vi "config_file_fgv.vi"(7 "cmd":enum16{"save", "load"}(ring), 8 "error in":errorcluster, 11 "Config":T1={"Lower Cut-Off"=0.5, "Vacuum Trigger level"=20.0, "state settings"={"method"=enum."histogram", "histogram size"=512, "histogram method"=enum."mode", "reserved"=1.0}, "SPA-300 Setting"={"Bonding force (g)"=0.0, "Bonding time (ms)"=512.0, "Pickup force (g)"=0.0, "Pickup time (ms)"=1.0, "Speed"=enum."Slow"}, "sensor file"=path ""} {"state settings"."reserved" format="%0.2f"}) -> (0 "error out":errorcluster, 2 "XML String":string caption="XML 문자열", 3 "var":T1={"Lower Cut-Off"=0.5, "Vacuum Trigger level"=20.0, "state settings"={"method"=enum."histogram", "histogram size"=512, "histogram method"=enum."mode", "reserved"=1.0}, "SPA-300 Setting"={"Bonding force (g)"=0.0, "Bonding time (ms)"=512.0, "Pickup force (g)"=0.0, "Pickup time (ms)"=1.0, "Speed"=enum."Slow"}, "sensor file"=path ""} {"state settings"."reserved" format="%0.2f"})   [LabVIEW 2016]
uses:
  ctl/config_ctl.ctl
  <vilib>/Utility/xml.llb/Write to XML File(string).vi
  <vilib>/Utility/xml.llb/Read From XML File(string).vi
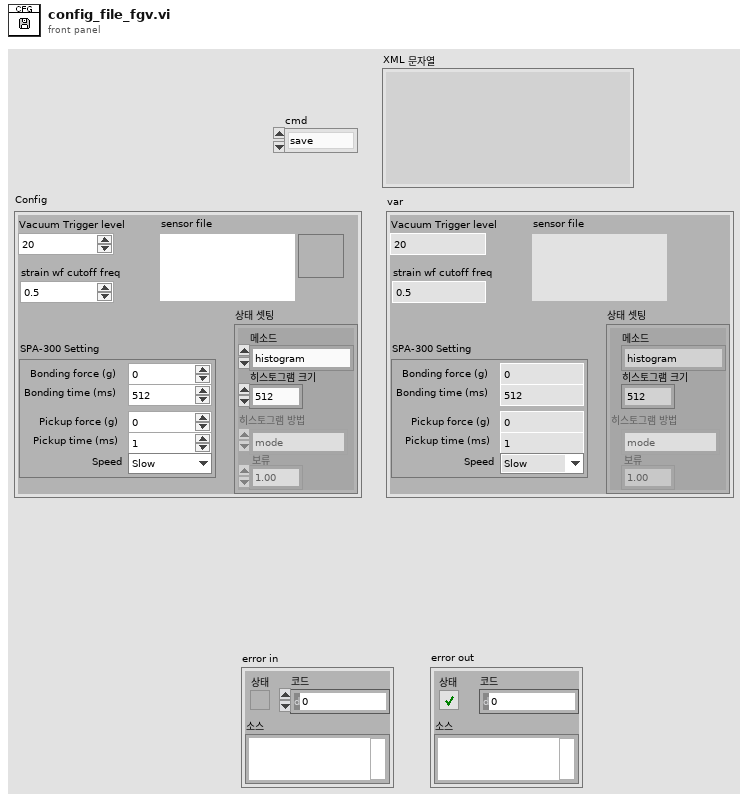
[diagram p1: front panel]
types:
  T1 = typedef "config_ctl.ctl" = cluster{"Lower Cut-Off":dbl, "Vacuum Trigger level":dbl, "state settings":cluster{"method":enum32{"histogram", "peak", "auto select"}, "histogram size":i32, "histogram method":enum16{"mode"}, "reserved":dbl}, "SPA-300 Setting":cluster{"Bonding force (g)":dbl, "Bonding time (ms)":dbl, "Pickup force (g)":dbl, "Pickup time (ms)":dbl, "Speed":enum16{"Slow", "Fast"}}, "sensor file":path}
  T2 = enum16{"open", "replace", "create", "open or create", "replace or create", "replace or create with confirmation"}
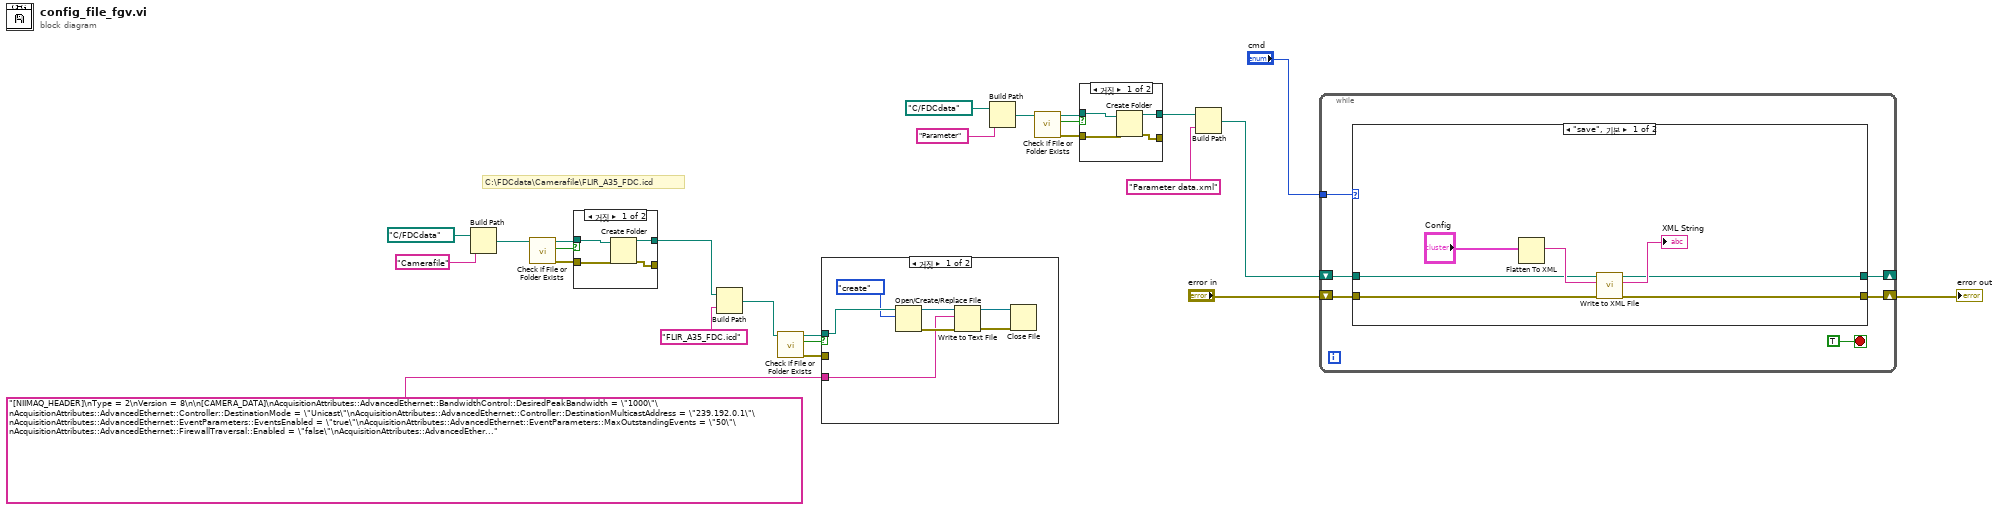
[diagram p0: block diagram]
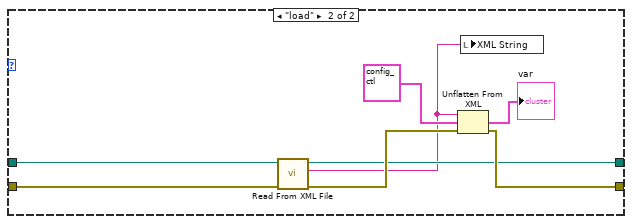
[diagram p5: hidden frame]
diagram:
  # "C:\\FDCdata\\Camerafile\\FLIR_A35_FDC.icd"
  n1 = Build Path(base path=path "C:/FDCdata" ("파일 경로(대화 상자 사용)"), name or relative path="Camerafile" ("이름 또는 상대 경로")) -> (appended path=w15:path)
  n2 = call <vilib>:"Check if File or Folder Exists.vi"("path"=w15) -> ("error out"=w14:errorcluster, "file or folder exists?"=w13:bool, "dup path"=w12:path)  [unwired: 8 in]
  n3 = case shown="거짓" w13 {
    tunnel: w12 -> [w29 w31]
    tunnel: w14 -> [w28 w30]
    tunnel: [w27 w31] -> w8
    tunnel: [w26 w30] -> _
    frame False {
      n4 = Create Folder(path (use dialog)=w29, error in=w28) -> (created path=w27:path, error out=w26:errorcluster)  [unwired: 1 in, 1 out]
    }
    frame True {
    }
  }
  n5 = Build Path(base path=w8, name or relative path="FLIR_A35_FDC.icd" ("이름 또는 상대 경로")) -> (appended path=w4:path)
  n6 = call <vilib>:"Check if File or Folder Exists.vi"("path"=w4) -> ("error out"=w5:errorcluster, "file or folder exists?"=w6:bool, "dup path"=w7:path)  [unwired: 8 in]
  n7 = case shown="거짓" w6 {
    tunnel: w7 -> [w38 _]
    tunnel: w5 -> [_ _]
    tunnel: "[NIIMAQ_HEADER]\nType = 2\nVersion = 8\n\n[CAMERA_DATA]\nAcquisitionAttributes::AdvancedEthernet::BandwidthControl::DesiredPeakBandwidth = \"1000\"\nAcquisitionAttributes::AdvancedEthernet::Controller::DestinationMode = \"Unicast\"\nAcquisitionAttributes::AdvancedEthernet::Controller::DestinationMulticastAddress = \"239.192.0.1\"\nAcquisitionAttributes::AdvancedEthernet::EventParameters::EventsEnabled = \"true\"\nAcquisitionAttributes::AdvancedEthernet::EventParameters::MaxOutstandingEvents = \"50\"\nAcquisitionAttributes::AdvancedEthernet::FirewallTraversal::Enabled = \"false\"\nAcquisitionAttributes::AdvancedEthernet::FirewallTraversal::KeepAliveTime = \"30\"\nAcquisitionAttributes::AdvancedEthernet::LostPacketMode = \"Ignore\"\nAcquisitionAttributes::AdvancedEthernet::ResendParameters::MaxResendsPerPacket = \"25\"\nAcquisitionAttributes::AdvancedEthernet::ResendParameters::MemoryWindowSize = \"1024\"\nAcquisitionAttributes::AdvancedEthernet::ResendParameters::MissingPacketTimeout = \"2\"\nAcquisitionAttributes::AdvancedEthernet::ResendParameters::NewPacketTimeout = \"100\"\nAcquisitionAttributes::AdvancedEthernet::ResendParameters::ResendBatchingPercentage = \"10\"\nAcquisitionAttributes::AdvancedEthernet::ResendParameters::ResendResponseTimeout = \"2\"\nAcquisitionAttributes::AdvancedEthernet::ResendParameters::ResendsEnabled = \"true\"\nAcquisitionAttributes::AdvancedEthernet::ResendParameters::ResendThresholdPercentage = \"5\"\nAcquisitionAttributes::AdvancedEthernet::ResendParameters::ResendTimerResolution = \"1\"\nAcquisitionAttributes::AdvancedEthernet::TestPacketParameters::MaxTestPacketRetries = \"1\"\nAcquisitionAttributes::AdvancedEthernet::TestPacketParameters::TestPacketEnabled = \"true\"\nAcquisitionAttributes::AdvancedEthernet::TestPacketParameters::TestPacketTimeout = \"250\"\nAcquisitionAttributes::AdvancedGenicam::CommandTimeout = \"100\"\nAcquisitionAttributes::Bayer::Algorithm = \"Bilinear\"\nAcquisitionAttributes::Bayer::GainB = \"1\"\nAcquisitionAttributes::Bayer::GainG = \"1\"\nAcquisitionAttributes::Bayer::GainR = \"1\"\nAcquisitionAttributes::Bayer::Pattern = \"Use hardware value\"\nAcquisitionAttributes::BitsPerPixel = \"Use hardware value\"\nAcquisitionAttributes::ChunkDataDecoding::ChunkDataDecodingEnabled = \"false\"\nAcquisitionAttributes::ChunkDataDecoding::MaximumChunkCopySize = \"64\"\nAcquisitionAttributes::IgnoreFirstFrame = \"false\"\nAcquisitionAttributes::ImageDecoderCopyMode = \"Auto\"\nAcquisitionAttributes::OutputImageType = \"Auto\"\nAcquisitionAttributes::OverwriteMode = \"Get Newest\"\nAcquisitionAttributes::PacketSize = \"1000\"\nAcquisitionAttributes::PixelSignedness = \"Signed\"\nAcquisitionAttributes::ReceiveTimestampMode = \"None\"\nAcquisitionAttributes::ShiftPixelBits = \"false\"\nAcquisitionAttributes::SwapPixelBytes = \"false\"\nAcquisitionAttributes::Timeout = \"5000\"\nCameraAttributes::AcquisitionControl::AcquisitionFrameCount = \"1\"\nCameraAttributes::AcquisitionControl::AcquisitionMode = \"Continuous\"\nCameraAttributes::CameraControl::BaudRate = \"baudAuto\"\nCameraAttributes::CameraControl::CorrectionMask = \"575\"\nCameraAttributes::CameraControl::IgnoreCRC = \"On\"\nCameraAttributes::CameraControl::NUCMode = \"Automatic\"\nCameraAttributes::CameraControl::SensorDDEIndex = \"17\"\nCameraAttributes::CameraControl::SensorDDEMode = \"Automatic\"\nCameraAttributes::CameraControl::SensorGainMode = \"LowGainMode\"\nCameraAttributes::CameraControl::ShutterPosition = \"Open\"\nCameraAttributes::CounterAndTimerControl::CounterSelector = \"Counter1\"\nCameraAttributes::CounterAndTimerControl::CounterDecrementEventSource = \"Off\"\nCameraAttributes::CounterAndTimerControl::CounterDuration = \"0\"\nCameraAttributes::CounterAndTimerControl::CounterEventSource = \"Off\"\nCameraAttributes::CounterAndTimerControl::CounterResetActivation = \"Off\"\nCameraAttributes::CounterAndTimerControl::CounterResetSource = \"PLC_Q3\"\nCameraAttributes::CounterAndTimerControl::CounterTriggerSource = \"Off\"\nCameraAttributes::CounterAndTimerControl::CounterValue = \"0\"\nCameraAttributes::CounterAndTimerControl::TimerSelector = \"Timer1\"\nCameraAttributes::CounterAndTimerControl::TimerDelayRaw = \"1024\"\nCameraAttributes::CounterAndTimerControl::TimerDurationRaw = \"4096\"\nCameraAttributes::CounterAndTimerControl::TimerGranularityFactor = \"0\"\nCameraAttributes::CounterAndTimerControl::TimerTriggerActivation = \"RisingEdge\"\nCameraAttributes::CounterAndTimerControl::TimerTriggerSource = \"PLC_Q\"\nCameraAttributes::CounterAndTimerControl::TimerSelector = \"Timer2\"\nCameraAttributes::CounterAndTimerControl::TimerDelayRaw = \"1024\"\nCameraAttributes::CounterAndTimerControl::TimerDurationRaw = \"4096\"\nCameraAttributes::CounterAndTimerControl::TimerGranularityFactor = \"0\"\nCameraAttributes::CounterAndTimerControl::TimerTriggerActivation = \"RisingEdge\"\nCameraAttributes::CounterAndTimerControl::TimerTriggerSource = \"PLC_Q\"\nCameraAttributes::CounterAndTimerControl::TimerSelector = \"Timer3\"\nCameraAttributes::CounterAndTimerControl::TimerDelayRaw = \"1024\"\nCameraAttributes::CounterAndTimerControl::TimerDurationRaw = \"4096\"\nCameraAttributes::CounterAndTimerControl::TimerGranularityFactor = \"0\"\nCameraAttributes::CounterAndTimerControl::TimerTriggerActivation = \"RisingEdge\"\nCameraAttributes::CounterAndTimerControl::TimerTriggerSource = \"PLC_Q\"\nCameraAttributes::CounterAndTimerControl::TimerSelector = \"Timer4\"\nCameraAttributes::CounterAndTimerControl::TimerDelayRaw = \"1024\"\nCameraAttributes::CounterAndTimerControl::TimerDurationRaw = \"4096\"\nCameraAttributes::CounterAndTimerControl::TimerGranularityFactor = \"0\"\nCameraAttributes::CounterAndTimerControl::TimerTriggerActivation = \"RisingEdge\"\nCameraAttributes::CounterAndTimerControl::TimerTriggerSource = \"PLC_Q\"\nCameraAttributes::CounterAndTimerControl::TimerSelector = \"Timer1\"\nCameraAttributes::DeviceControl::DeviceScanType = \"Areascan\"\nCameraAttributes::DigitalIOControl::LineSelector = \"Line0\"\nCameraAttributes::DigitalIOControl::LineDebounceFactor = \"0\"\nCameraAttributes::DigitalIOControl::SyncMode = \"Disabled\"\nCameraAttributes::DigitalIOControl::UserOutputSelector = \"UserOutput0\"\nCameraAttributes::DigitalIOControl::UserOutputValue = \"true\"\nCameraAttributes::EventControl::EventSelector = \"PLC_Interrupt_FIFO0_Q15\"\nCameraAttributes::EventControl::EventNotification = \"On\"\nCameraAttributes::EventControl::EventSelector = \"PLC_Interrupt_FIFO0_Q3\"\nCameraAttributes::EventControl::EventNotification = \"Off\"\nCameraAttributes::EventControl::EventSelector = \"PLC_Interrupt_FIFO0_Q7\"\nCameraAttributes::EventControl::EventNotification = \"Off\"\nCameraAttributes::EventControl::EventSelector = \"PLC_Interrupt_FIFO0_Q10\"\nCameraAttributes::EventControl::EventNotification = \"Off\"\nCameraAttributes::EventControl::EventSelector = \"IPEngineCamHeadSerialComLog\"\nCameraAttributes::EventControl::EventNotification = \"Off\"\nCameraAttributes::EventControl::EventSelector = \"IPEngineCamHeadSerialComLog\"\nCameraAttributes::ImageFormatControl::BinningHorizontal = \"1\"\nCameraAttributes::ImageFormatControl::BinningVertical = \"1\"\nCameraAttributes::ImageFormatControl::DecimationHorizontal = \"1\"\nCameraAttributes::ImageFormatControl::DecimationVertical = \"1\"\nCameraAttributes::ImageFormatControl::Height = \"256\"\nCameraAttributes::ImageFormatControl::OffsetX = \"0\"\nCameraAttributes::ImageFormatControl::OffsetY = \"0\"\nCameraAttributes::ImageFormatControl::PixelFormat = \"Mono16\"\nCameraAttributes::ImageFormatControl::SensorDigitizationTaps = \"One\"\nCameraAttributes::ImageFormatControl::TestImageSelector = \"Off\"\nCameraAttributes::ImageFormatControl::Width = \"320\"\nCameraAttributes::ImageStreamControl::CMOSBitDepth = \"bit14bit\"\nCameraAttributes::ImageStreamControl::DigitalOutput = \"bit14bit\"\nCameraAttributes::ImageStreamControl::IRTestPattern = \"Off\"\nCameraAttributes::ImageStreamControl::LVDSBitDepth = \"bit14bit\"\nCameraAttributes::ImageStreamControl::LVDSMode = \"Disabled\"\nCameraAttributes::ImageStreamControl::XPMode = \"CMOS\"\nCameraAttributes::IPEngine::Grabber::Channel0::AcquisitionConfiguration::GrbCh0AcqCfgIncludeMetadataInImage = \"false\"\nCameraAttributes::IPEngine::Grabber::Channel0::AcquisitionConfiguration::GrbCh0AcqCfgInvertPixelData = \"false\"\nCameraAttributes::IPEngine::Grabber::Channel0::AcquisitionConfiguration::GrbCh0AcqCfgMemoryWaterLevel = \"Level75\"\nCameraAttributes::IPEngine::Grabber::Channel0::AcquisitionConfiguration::GrbCh0AcqCfgPixelBusDataPortMapping = \"CBA\"\nCameraAttributes::IPEngine::Grabber::Channel0::TriggerConfiguration::GrbCh0TrigCfgAutomaticInternalRetrigger = \"false\"\nCameraAttributes::IPEngine::Grabber::Channel0::TriggerConfiguration::GrbCh0TrigCfgContinuousPipeCount = \"Two\"\nCameraAttributes::IPEngine::Grabber::Channel0::TriggerConfiguration::GrbCh0TrigCfgFrameToSkip = \"0\"\nCameraAttributes::IPEngine::Grabber::Channel0::TriggerConfiguration::GrbCh0TrigCfgPLCTriggerable = \"false\"\nCameraAttributes::IPEngine::Grabber::Channel0Extension::GrabberMetadata::GrbCh0MetadataInsertionMode = \"FirstFourBytesOfFirstAcquiredLine\"\nCameraAttributes::IPEngine::Grabber::Channel0Extension::GrabberMetadata::GrbCh0MetadataMsbOverride = \"NotOverriden\"\nCameraAttributes::IPEngine::Grabber::Channel0Extension::GrabberMetadata::GrbCh0MetadataSourceSelection = \"BlockID\"\nCameraAttributes::IPEngine::PortCommunication::Uart0::Uart0BaudRate = \"Baud57600\"\nCameraAttributes::IPEngine::PortCommunication::Uart0::Uart0BaudRateFactor = \"1\"\nCameraAttributes::IPEngine::PortCommunication::Uart0::Uart0BreakDetection = \"true\"\nCameraAttributes::IPEngine::PortCommunication::Uart0::Uart0BreakGeneration = \"true\"\nCameraAttributes::IPEngine::PortCommunication::Uart0::Uart0Loopback = \"false\"\nCameraAttributes::IPEngine::PortCommunication::Uart0::Uart0NumOfStopBits = \"One\"\nCameraAttributes::IPEngine::PortCommunication::Uart0::Uart0Parity = \"None\"\nCameraAttributes::IPEngine::PortCommunication::Uart0::Uart0ReadyToReceive = \"true\"\nCameraAttributes::IPEngine::PortCommunication::Uart1::Uart1BaudRate = \"Baud9600\"\nCameraAttributes::IPEngine::PortCommunication::Uart1::Uart1BaudRateFactor = \"1\"\nCameraAttributes::IPEngine::PortCommunication::Uart1::Uart1BreakDetection = \"false\"\nCameraAttributes::IPEngine::PortCommunication::Uart1::Uart1BreakGeneration = \"false\"\nCameraAttributes::IPEngine::PortCommunication::Uart1::Uart1Loopback = \"false\"\nCameraAttributes::IPEngine::PortCommunication::Uart1::Uart1NumOfStopBits = \"One\"\nCameraAttributes::IPEngine::PortCommunication::Uart1::Uart1Parity = \"None\"\nCameraAttributes::IPEngine::PortCommunication::Uart1::Uart1ReadyToReceive = \"false\"\nCameraAttributes::IPEngine::ProgrammableLogicController::ControlBits::PLC_ctrl0 = \"true\"\nCameraAttributes::IPEngine::ProgrammableLogicController::ControlBits::PLC_ctrl1 = \"false\"\nCameraAttributes::IPEngine::ProgrammableLogicController::ControlBits::PLC_ctrl2 = \"false\"\nCameraAttributes::IPEngine::ProgrammableLogicController::ControlBits::PLC_ctrl3 = \"false\"\nCameraAttributes::IPEngine::ProgrammableLogicController::EnhancedFunctionBlock::CounterTriggerGenerator::PLC_ts_trig0_Enable = \"false\"\nCameraAttributes::IPEngine::ProgrammableLogicController::EnhancedFunctionBlock::CounterTriggerGenerator::PLC_ts_trig1_Enable = \"false\"\nCameraAttributes::IPEngine::ProgrammableLogicController::EnhancedFunctionBlock::CounterTriggerGenerator::PLC_ts_trig2_Enable = \"false\"\nCameraAttributes::IPEngine::ProgrammableLogicController::EnhancedFunctionBlock::CounterTriggerGenerator::PLC_ts_trig3_Enable = \"false\"\nCameraAttributes::IPEngine::ProgrammableLogicController::EnhancedFunctionBlock::CounterTriggerGenerator::PLC_ts_trig_CounterSelect = \"GevTimestampValueLow\"\nCameraAttributes::IPEngine::ProgrammableLogicController::EnhancedFunctionBlock::CounterTriggerGenerator::PLC_ts_trig_Time = \"0\"\nCameraAttributes::IPEngine::ProgrammableLogicController::EnhancedFunctionBlock::Delayer0::PLC_del0_DelayCount = \"1\"\nCameraAttributes::IPEngine::ProgrammableLogicController::EnhancedFunctionBlock::Delayer0::PLC_del0_InputSignal = \"PLC_Q3\"\nCameraAttributes::IPEngine::ProgrammableLogicController::EnhancedFunctionBlock::Delayer0::PLC_del0_ReferenceTimingSignal = \"PLC_rsl0_out\"\nCameraAttributes::IPEngine::ProgrammableLogicController::EnhancedFunctionBlock::Rescaler0::PLC_rsl0_BackupEnabled = \"false\"\nCameraAttributes::IPEngine::ProgrammableLogicController::EnhancedFunctionBlock::Rescaler0::PLC_rsl0_BackupInputSignal = \"Timer1Out\"\nCameraAttributes::IPEngine::ProgrammableLogicController::EnhancedFunctionBlock::Rescaler0::PLC_rsl0_BackupSwitchoverDelay = \"0\"\nCameraAttributes::IPEngine::ProgrammableLogicController::EnhancedFunctionBlock::Rescaler0::PLC_rsl0_Divider = \"256\"\nCameraAttributes::IPEngine::ProgrammableLogicController::EnhancedFunctionBlock::Rescaler0::PLC_rsl0_Granularity = \"OneSystemClockCycle\"\nCameraAttributes::IPEngine::ProgrammableLogicController::EnhancedFunctionBlock::Rescaler0::PLC_rsl0_InputSignal = \"PLC_Q3\"\nCameraAttributes::IPEngine::ProgrammableLogicController::EnhancedFunctionBlock::Rescaler0::PLC_rsl0_Multiplier = \"FrequencyX256\"\nCameraAttributes::IPEngine::ProgrammableLogicController::LookupTable::Q0::PLC_Q0_Operator0 = \"Or\"\nCameraAttributes::IPEngine::ProgrammableLogicController::LookupTable::Q0::PLC_Q0_Operator1 = \"Or\"\nCameraAttributes::IPEngine::ProgrammableLogicController::LookupTable::Q0::PLC_Q0_Operator2 = \"Or\"\nCameraAttributes::IPEngine::ProgrammableLogicController::LookupTable::Q0::PLC_Q0_Variable0 = \"PLC_I5\"\nCameraAttributes::IPEngine::ProgrammableLogicController::LookupTable::Q0::PLC_Q0_Variable1 = \"Zero\"\nCameraAttributes::IPEngine::ProgrammableLogicController::LookupTable::Q0::PLC_Q0_Variable2 = \"Zero\"\nCameraAttributes::IPEngine::ProgrammableLogicController::LookupTable::Q0::PLC_Q0_Variable3 = \"Zero\"\nCameraAttributes::IPEngine::ProgrammableLogicController::LookupTable::Q10::PLC_Q10_Operator0 = \"Or\"\nCameraAttributes::IPEngine::ProgrammableLogicController::LookupTable::Q10::PLC_Q10_Operator1 = \"Or\"\nCameraAttributes::IPEngine::ProgrammableLogicController::LookupTable::Q10::PLC_Q10_Operator2 = \"Or\"\nCameraAttributes::IPEngine::ProgrammableLogicController::LookupTable::Q10::PLC_Q10_Variable0 = \"Zero\"\nCameraAttributes::IPEngine::ProgrammableLogicController::LookupTable::Q10::PLC_Q10_Variable1 = \"Zero\"\nCameraAttributes::IPEngine::ProgrammableLogicController::LookupTable::Q10::PLC_Q10_Variable2 = \"Zero\"\nCameraAttributes::IPEngine::ProgrammableLogicController::LookupTable::Q10::PLC_Q10_Variable3 = \"Zero\"\nCameraAttributes::IPEngine::ProgrammableLogicController::LookupTable::Q11::PLC_Q11_Operator0 = \"Or\"\nCameraAttributes::IPEngine::ProgrammableLogicController::LookupTable::Q11::PLC_Q11_Operator1 = \"Or\"\nCameraAttributes::IPEngine::ProgrammableLogicController::LookupTable::Q11::PLC_Q11_Operator2 = \"Or\"\nCameraAttributes::IPEngine::ProgrammableLogicController::LookupTable::Q11::PLC_Q11_Variable0 = \"Zero\"\nCameraAttributes::IPEngine::ProgrammableLogicController::LookupTable::Q11::PLC_Q11_Variable1 = \"Zero\"\nCameraAttributes::IPEngine::ProgrammableLogicController::LookupTable::Q11::PLC_Q11_Variable2 = \"Zero\"\nCameraAttributes::IPEngine::ProgrammableLogicController::LookupTable::Q11::PLC_Q11_Variable3 = \"Zero\"\nCameraAttributes::IPEngine::ProgrammableLogicController::LookupTable::Q12::PLC_Q12_Operator0 = \"Or\"\nCameraAttributes::IPEngine::ProgrammableLogicController::LookupTable::Q12::PLC_Q12_Operator1 = \"Or\"\nCameraAttributes::IPEngine::ProgrammableLogicController::LookupTable::Q12::PLC_Q12_Operator2 = \"Or\"\nCameraAttributes::IPEngine::ProgrammableLogicController::LookupTable::Q12::PLC_Q12_Variable0 = \"Zero\"\nCameraAttributes::IPEngine::ProgrammableLogicController::LookupTable::Q12::PLC_Q12_Variable1 = \"Zero\"\nCameraAttributes::IPEngine::ProgrammableLogicController::LookupTable::Q12::PLC_Q12_Variable2 = \"Zero\"\nCameraAttributes::IPEngine::ProgrammableLogicController::LookupTable::Q12::PLC_Q12_Variable3 = \"Zero\"\nCameraAttributes::IPEngine::ProgrammableLogicController::LookupTable::Q13::PLC_Q13_Operator0 = \"Or\"\nCameraAttributes::IPEngine::ProgrammableLogicController::LookupTable::Q13::PLC_Q13_Operator1 = \"Or\"\nCameraAttributes::IPEngine::ProgrammableLogicController::LookupTable::Q13::PLC_Q13_Operator2 = \"Or\"\nCameraAttributes::IPEngine::ProgrammableLogicController::LookupTable::Q13::PLC_Q13_Variable0 = \"Zero\"\nCameraAttributes::IPEngine::ProgrammableLogicController::LookupTable::Q13::PLC_Q13_Variable1 = \"Zero\"\nCameraAttributes::IPEngine::ProgrammableLogicController::LookupTable::Q13::PLC_Q13_Variable2 = \"Zero\"\nCameraAttributes::IPEngine::ProgrammableLogicController::LookupTable::Q13::PLC_Q13_Variable3 = \"Zero\"\nCameraAttributes::IPEngine::ProgrammableLogicController::LookupTable::Q14::PLC_Q14_Operator0 = \"Or\"\nCameraAttributes::IPEngine::ProgrammableLogicController::LookupTable::Q14::PLC_Q14_Operator1 = \"Or\"\nCameraAttributes::IPEngine::ProgrammableLogicController::LookupTable::Q14::PLC_Q14_Operator2 = \"Or\"\nCameraAttributes::IPEngine::ProgrammableLogicController::LookupTable::Q14::PLC_Q14_Variable0 = \"Zero\"\nCameraAttributes::IPEngine::ProgrammableLogicController::LookupTable::Q14::PLC_Q14_Variable1 = \"Zero\"\nCameraAttributes::IPEngine::ProgrammableLogicController::LookupTable::Q14::PLC_Q14_Variable2 = \"Zero\"\nCameraAttributes::IPEngine::ProgrammableLogicController::LookupTable::Q14::PLC_Q14_Variable3 = \"Zero\"\nCameraAttributes::IPEngine::ProgrammableLogicController::LookupTable::Q15::PLC_Q15_Operator0 = \"Or\"\nCameraAttributes::IPEngine::ProgrammableLogicController::LookupTable::Q15::PLC_Q15_Operator1 = \"Or\"\nCameraAttributes::IPEngine::ProgrammableLogicController::LookupTable::Q15::PLC_Q15_Operator2 = \"Or\"\nCameraAttributes::IPEngine::ProgrammableLogicController::LookupTable::Q15::PLC_Q15_Variable0 = \"Zero\"\nCameraAttributes::IPEngine::ProgrammableLogicController::LookupTable::Q15::PLC_Q15_Variable1 = \"Zero\"\nCameraAttributes::IPEngine::ProgrammableLogicController::LookupTable::Q15::PLC_Q15_Variable2 = \"Zero\"\nCameraAttributes::IPEngine::ProgrammableLogicController::LookupTable::Q15::PLC_Q15_Variable3 = \"Zero\"\nCameraAttributes::IPEngine::ProgrammableLogicController::LookupTable::Q16::PLC_Q16_Operator0 = \"Or\"\nCameraAttributes::IPEngine::ProgrammableLogicController::LookupTable::Q16::PLC_Q16_Operator1 = \"Or\"\nCameraAttributes::IPEngine::ProgrammableLogicController::LookupTable::Q16::PLC_Q16_Operator2 = \"Or\"\nCameraAttributes::IPEngine::ProgrammableLogicController::LookupTable::Q16::PLC_Q16_Variable0 = \"Zero\"\nCameraAttributes::IPEngine::ProgrammableLogicController::LookupTable::Q16::PLC_Q16_Variable1 = \"Zero\"\nCameraAttributes::IPEngine::ProgrammableLogicController::LookupTable::Q16::PLC_Q16_Variable2 = \"Zero\"\nCameraAttributes::IPEngine::ProgrammableLogicController::LookupTable::Q16::PLC_Q16_Variable3 = \"Zero\"\nCameraAttributes::IPEngine::ProgrammableLogicController::LookupTable::Q17::PLC_Q17_Operator0 = \"Or\"\nCameraAttributes::IPEngine::ProgrammableLogicController::LookupTable::Q17::PLC_Q17_Operator1 = \"Or\"\nCameraAttributes::IPEngine::ProgrammableLogicController::LookupTable::Q17::PLC_Q17_Operator2 = \"Or\"\nCameraAttributes::IPEngine::ProgrammableLogicController::LookupTable::Q17::PLC_Q17_Variable0 = \"Zero\"\nCameraAttributes::IPEngine::ProgrammableLogicController::LookupTable::Q17::PLC_Q17_Variable1 = \"Zero\"\nCameraAttributes::IPEngine::ProgrammableLogicController::LookupTable::Q17::PLC_Q17_Variable2 = \"Zero\"\nCameraAttributes::IPEngine::ProgrammableLogicController::LookupTable::Q17::PLC_Q17_Variable3 = \"Zero\"\nCameraAttributes::IPEngine::ProgrammableLogicController::LookupTable::Q1::PLC_Q1_Operator0 = \"Or\"\nCameraAttributes::IPEngine::ProgrammableLogicController::LookupTable::Q1::PLC_Q1_Operator1 = \"Or\"\nCameraAttributes::IPEngine::ProgrammableLogicController::LookupTable::Q1::PLC_Q1_Operator2 = \"Or\"\nCameraAttributes::IPEngine::ProgrammableLogicController::LookupTable::Q1::PLC_Q1_Variable0 = \"Zero\"\nCameraAttributes::IPEngine::ProgrammableLogicController::LookupTable::Q1::PLC_Q1_Variable1 = \"Zero\"\nCameraAttributes::IPEngine::ProgrammableLogicController::LookupTable::Q1::PLC_Q1_Variable2 = \"Zero\"\nCameraAttributes::IPEngine::ProgrammableLogicController::LookupTable::Q1::PLC_Q1_Variable3 = \"Zero\"\nCameraAttributes::IPEngine::ProgrammableLogicController::LookupTable::Q2::PLC_Q2_Operator0 = \"Or\"\nCameraAttributes::IPEngine::ProgrammableLogicController::LookupTable::Q2::PLC_Q2_Operator1 = \"Or\"\nCameraAttributes::IPEngine::ProgrammableLogicController::LookupTable::Q2::PLC_Q2_Operator2 = \"Or\"\nCameraAttributes::IPEngine::ProgrammableLogicController::LookupTable::Q2::PLC_Q2_Variable0 = \"PLC_I1\"\nCameraAttributes::IPEngine::ProgrammableLogicController::LookupTable::Q2::PLC_Q2_Variable1 = \"Zero\"\nCameraAttributes::IPEngine::ProgrammableLogicController::LookupTable::Q2::PLC_Q2_Variable2 = \"Zero\"\nCameraAttributes::IPEngine::ProgrammableLogicController::LookupTable::Q2::PLC_Q2_Variable3 = \"Zero\"\nCameraAttributes::IPEngine::ProgrammableLogicController::LookupTable::Q3::PLC_Q3_Operator0 = \"Or\"\nCameraAttributes::IPEngine::ProgrammableLogicController::LookupTable::Q3::PLC_Q3_Operator1 = \"Or\"\nCameraAttributes::IPEngine::ProgrammableLogicController::LookupTable::Q3::PLC_Q3_Operator2 = \"Or\"\nCameraAttributes::IPEngine::ProgrammableLogicController::LookupTable::Q3::PLC_Q3_Variable0 = \"One\"\nCameraAttributes::IPEngine::ProgrammableLogicController::LookupTable::Q3::PLC_Q3_Variable1 = \"Zero\"\nCameraAttributes::IPEngine::ProgrammableLogicController::LookupTable::Q3::PLC_Q3_Variable2 = \"Zero\"\nCameraAttributes::IPEngine::ProgrammableLogicController::LookupTable::Q3::PLC_Q3_Variable3 = \"Zero\"\nCameraAttributes::IPEngine::ProgrammableLogicController::LookupTable::Q4::PLC_Q4_Operator0 = \"Or\"\nCameraAttributes::IPEngine::ProgrammableLogicController::LookupTable::Q4::PLC_Q4_Operator1 = \"Or\"\nCameraAttributes::IPEngine::ProgrammableLogicController::LookupTable::Q4::PLC_Q4_Operator2 = \"Or\"\nCameraAttributes::IPEngine::ProgrammableLogicController::LookupTable::Q4::PLC_Q4_Variable0 = \"Zero\"\nCameraAttributes::IPEngine::ProgrammableLogicController::LookupTable::Q4::PLC_Q4_Variable1 = \"Zero\"\nCameraAttributes::IPEngine::ProgrammableLogicController::LookupTable::Q4::PLC_Q4_Variable2 = \"Zero\"\nCameraAttributes::IPEngine::ProgrammableLogicController::LookupTable::Q4::PLC_Q4_Variable3 = \"Zero\"\nCameraAttributes::IPEngine::ProgrammableLogicController::LookupTable::Q5::PLC_Q5_Operator0 = \"Or\"\nCameraAttributes::IPEngine::ProgrammableLogicController::LookupTable::Q5::PLC_Q5_Operator1 = \"Or\"\nCameraAttributes::IPEngine::ProgrammableLogicController::LookupTable::Q5::PLC_Q5_Operator2 = \"Or\"\nCameraAttributes::IPEngine::ProgrammableLogicController::LookupTable::Q5::PLC_Q5_Variable0 = \"Zero\"\nCameraAttributes::IPEngine::ProgrammableLogicController::LookupTable::Q5::PLC_Q5_Variable1 = \"Zero\"\nCameraAttributes::IPEngine::ProgrammableLogicController::LookupTable::Q5::PLC_Q5_Variable2 = \"Zero\"\nCameraAttributes::IPEngine::ProgrammableLogicController::LookupTable::Q5::PLC_Q5_Variable3 = \"Zero\"\nCameraAttributes::IPEngine::ProgrammableLogicController::LookupTable::Q6::PLC_Q6_Operator0 = \"Or\"\nCameraAttributes::IPEngine::ProgrammableLogicController::LookupTable::Q6::PLC_Q6_Operator1 = \"Or\"\nCameraAttributes::IPEngine::ProgrammableLogicController::LookupTable::Q6::PLC_Q6_Operator2 = \"Or\"\nCameraAttributes::IPEngine::ProgrammableLogicController::LookupTable::Q6::PLC_Q6_Variable0 = \"Zero\"\nCameraAttributes::IPEngine::ProgrammableLogicController::LookupTable::Q6::PLC_Q6_Variable1 = \"Zero\"\nCameraAttributes::IPEngine::ProgrammableLogicController::LookupTable::Q6::PLC_Q6_Variable2 = \"Zero\"\nCameraAttributes::IPEngine::ProgrammableLogicController::LookupTable::Q6::PLC_Q6_Variable3 = \"Zero\"\nCameraAttributes::IPEngine::ProgrammableLogicController::LookupTable::Q7::PLC_Q7_Operator0 = \"Or\"\nCameraAttributes::IPEngine::ProgrammableLogicController::LookupTable::Q7::PLC_Q7_Operator1 = \"Or\"\nCameraAttributes::IPEngine::ProgrammableLogicController::LookupTable::Q7::PLC_Q7_Operator2 = \"Or\"\nCameraAttributes::IPEngine::ProgrammableLogicController::LookupTable::Q7::PLC_Q7_Variable0 = \"Zero\"\nCameraAttributes::IPEngine::ProgrammableLogicController::LookupTable::Q7::PLC_Q7_Variable1 = \"Zero\"\nCameraAttributes::IPEngine::ProgrammableLogicController::LookupTable::Q7::PLC_Q7_Variable2 = \"Zero\"\nCameraAttributes::IPEngine::ProgrammableLogicController::LookupTable::Q7::PLC_Q7_Variable3 = \"Zero\"\nCameraAttributes::IPEngine::ProgrammableLogicController::LookupTable::Q8::PLC_Q8_Operator0 = \"Or\"\nCameraAttributes::IPEngine::ProgrammableLogicController::LookupTable::Q8::PLC_Q8_Operator1 = \"Or\"\nCameraAttributes::IPEngine::ProgrammableLogicController::LookupTable::Q8::PLC_Q8_Operator2 = \"Or\"\nCameraAttributes::IPEngine::ProgrammableLogicController::LookupTable::Q8::PLC_Q8_Variable0 = \"Zero\"\nCameraAttributes::IPEngine::ProgrammableLogicController::LookupTable::Q8::PLC_Q8_Variable1 = \"Zero\"\nCameraAttributes::IPEngine::ProgrammableLogicController::LookupTable::Q8::PLC_Q8_Variable2 = \"Zero\"\nCameraAttributes::IPEngine::ProgrammableLogicController::LookupTable::Q8::PLC_Q8_Variable3 = \"Zero\"\nCameraAttributes::IPEngine::ProgrammableLogicController::LookupTable::Q9::PLC_Q9_Operator0 = \"Or\"\nCameraAttributes::IPEngine::ProgrammableLogicController::LookupTable::Q9::PLC_Q9_Operator1 = \"Or\"\nCameraAttributes::IPEngine::ProgrammableLogicController::LookupTable::Q9::PLC_Q9_Operator2 = \"Or\"\nCameraAttributes::IPEngine::ProgrammableLogicController::LookupTable::Q9::PLC_Q9_Variable0 = \"Zero\"\nCameraAttributes::IPEngine::ProgrammableLogicController::LookupTable::Q9::PLC_Q9_Variable1 = \"Zero\"\nCameraAttributes::IPEngine::ProgrammableLogicController::LookupTable::Q9::PLC_Q9_Variable2 = \"Zero\"\nCameraAttributes::IPEngine::ProgrammableLogicController::LookupTable::Q9::PLC_Q9_Variable3 = \"Zero\"\nCameraAttributes::IPEngine::ProgrammableLogicController::PLCSpecialConfigurations::Line0Configuration = \"Zero\"\nCameraAttributes::IPEngine::ProgrammableLogicController::PLCSpecialConfigurations::Line1Configuration = \"Zero\"\nCameraAttributes::IPEngine::ProgrammableLogicController::PLCSpecialConfigurations::Line2Configuration = \"Zero\"\nCameraAttributes::IPEngine::ProgrammableLogicController::PLCSpecialConfigurations::Line3Configuration = \"Zero\"\nCameraAttributes::IPEngine::ProgrammableLogicController::PLCSpecialConfigurations::PLC_Q0_Configuration = \"Zero\"\nCameraAttributes::IPEngine::ProgrammableLogicController::PLCSpecialConfigurations::PLC_Q1_Configuration = \"Zero\"\nCameraAttributes::IPEngine::ProgrammableLogicController::PLCSpecialConfigurations::PLC_Q2_Configuration = \"Zero\"\nCameraAttributes::IPEngine::ProgrammableLogicController::PLCSpecialConfigurations::PLC_Q3_Configuration = \"Zero\"\nCameraAttributes::IPEngine::ProgrammableLogicController::PLCSpecialConfigurations::PLC_Q4_Configuration = \"Zero\"\nCameraAttributes::IPEngine::ProgrammableLogicController::PLCSpecialConfigurations::PLC_Q5_Configuration = \"Zero\"\nCameraAttributes::IPEngine::ProgrammableLogicController::PLCSpecialConfigurations::PLC_Q6_Configuration = \"Zero\"\nCameraAttributes::IPEngine::ProgrammableLogicController::PLCSpecialConfigurations::PLC_Q7_Configuration = \"Zero\"\nCameraAttributes::IPEngine::ProgrammableLogicController::SignalRoutingBlock::PLC_I0 = \"Line0\"\nCameraAttributes::IPEngine::ProgrammableLogicController::SignalRoutingBlock::PLC_I1 = \"Line1\"\nCameraAttributes::IPEngine::ProgrammableLogicController::SignalRoutingBlock::PLC_I2 = \"Line2\"\nCameraAttributes::IPEngine::ProgrammableLogicController::SignalRoutingBlock::PLC_I3 = \"Line3\"\nCameraAttributes::IPEngine::ProgrammableLogicController::SignalRoutingBlock::PLC_I4 = \"PLC_ctrl1\"\nCameraAttributes::IPEngine::ProgrammableLogicController::SignalRoutingBlock::PLC_I5 = \"PLC_ctrl0\"\nCameraAttributes::IPEngine::ProgrammableLogicController::SignalRoutingBlock::PLC_I6 = \"Timer2Out\"\nCameraAttributes::IPEngine::ProgrammableLogicController::SignalRoutingBlock::PLC_I7 = \"Timer1Out\"\nCameraAttributes::Measurement::B = \"1470\"\nCameraAttributes::Measurement::BInternal = \"1470000\"\nCameraAttributes::Measurement::F = \"1\"\nCameraAttributes::Measurement::FInternal = \"1000\"\nCameraAttributes::Measurement::FLens0 = \"1.24999999488\"\nCameraAttributes::Measurement::FLens1 = \"1.24999999488\"\nCameraAttributes::Measurement::FLensInternal0 = \"10240\"\nCameraAttributes::Measurement::FLensInternal1 = \"10240\"\nCameraAttributes::Measurement::FNumber = \"1.24999999488\"\nCameraAttributes::Measurement::J1 = \"3.01220703125\"\nCameraAttributes::Measurement::J1Internal = \"24676\"\nCameraAttributes::Measurement::LensNumber = \"Lens0\"\nCameraAttributes::Measurement::LensSelector = \"Lens0\"\nCameraAttributes::Measurement::FLens = \"10240\"\nCameraAttributes::Measurement::TauLens = \"5898\"\nCameraAttributes::Measurement::LensSelector = \"Lens1\"\nCameraAttributes::Measurement::FLens = \"10240\"\nCameraAttributes::Measurement::TauLens = \"5898\"\nCameraAttributes::Measurement::OInt = \"806\"\nCameraAttributes::Measurement::OInternal = \"806000\"\nCameraAttributes::Measurement::R = \"55768\"\nCameraAttributes::Measurement::TauLens0 = \"0.71997070017600007\"\nCameraAttributes::Measurement::TauLens1 = \"0.71997070017600007\"\nCameraAttributes::Measurement::TauLensInternal0 = \"5898\"\nCameraAttributes::Measurement::TauLensInternal1 = \"5898\"\nCameraAttributes::Measurement::TemperatureLinearMode = \"On\"\nCameraAttributes::Measurement::TemperatureLinearResolution = \"High\"\nCameraAttributes::Measurement::Transmission = \"0.71997070017600007\"\nCameraAttributes::Mono8VideoControl::ImageAdjustMethod = \"PlateauHistogram\"\nCameraAttributes::Mono8VideoControl::ITTFilter = \"64\"\nCameraAttributes::Mono8VideoControl::ITTMidpoint = \"127\"\nCameraAttributes::Mono8VideoControl::MaxAGCGain = \"6\"\nCameraAttributes::Mono8VideoControl::PlateauLevel = \"150\"\nCameraAttributes::Mono8VideoControl::SensorVideoStandard = \"NTSC60HZ\"\nCameraAttributes::Mono8VideoControl::VideoOrientation = \"Normal\"\nCameraAttributes::ObjectParameters::AtmosphericTemperature = \"295.14999999999998\"\nCameraAttributes::ObjectParameters::AtmosphericTransmission = \"0.99999999590400002\"\nCameraAttributes::ObjectParameters::AtmTaoInternal = \"8192\"\nCameraAttributes::ObjectParameters::AtmTempInternal = \"2200\"\nCameraAttributes::ObjectParameters::EmissInternal = \"8192\"\nCameraAttributes::ObjectParameters::ObjectEmissivity = \"0.99999999590400002\"\nCameraAttributes::ObjectParameters::ReflectedTemperature = \"295.14999999999998\"\nCameraAttributes::ObjectParameters::ReflectedTempInternal = \"2200\"\nCameraAttributes::ObjectParameters::WindowTaoInternal = \"8192\"\nCameraAttributes::ObjectParameters::WindowTemperature = \"295.14999999999998\"\nCameraAttributes::ObjectParameters::WindowTempInternal = \"2200\"\nCameraAttributes::ObjectParameters::WindowTransmission = \"0.99999999590400002\"\nCameraAttributes::TransportLayerControl::GevSupportedOptionSelector = \"IPConfigurationLLA\"\nCameraAttributes::TransportLayerControl::GevTimestampCounterSelector = \"GevTimestamp\"\nCameraAttributes::TransportLayerControl::GevTimestampResetActivation = \"Disabled\"\nCameraAttributes::TransportLayerControl::GevTimestampResetSource = \"PLC_Q3\"\nCameraAttributes::TransportLayerControl::GevTimestampSetActivation = \"Disabled\"\nCameraAttributes::TransportLayerControl::GevTimestampSetSource = \"PLC_Q3\"\nCameraAttributes::TransportLayerControl::GevTimestampValueAtSet = \"0\"\n" -> [w32 _]
    frame False {
      n8 = Open/Create/Replace File(file path (use dialog)=w38, operation (0:open)=T2."create" ("동작(0:open)")) -> (refnum out=w35:refnum<file>, error out=w36:errorcluster)  [unwired: 4 in, 1 out]
      n9 = Write to Text File(file (use dialog)=w35, text=w32, error in=w36) -> (refnum out=w34:refnum<file>, error out=w33:errorcluster)  [unwired: 1 in, 1 out]
      n10 = Close File(refnum=w34, error in=w33) -> ()  [unwired: 2 out]
    }
    frame True {
    }
  }
  n11 = Build Path(base path=path "C:/FDCdata" ("파일 경로(대화 상자 사용)"), name or relative path="Parameter" ("이름 또는 상대 경로")) -> (appended path=w19:path)
  n12 = call <vilib>:"Check if File or Folder Exists.vi"("path"=w19) -> ("error out"=w20:errorcluster, "file or folder exists?"=w21:bool, "dup path"=w22:path)  [unwired: 8 in]
  n13 = case shown="거짓" w21 {
    tunnel: w22 -> [w42 w44]
    tunnel: w20 -> [w41 w43]
    tunnel: [w40 w44] -> w17
    tunnel: [w39 w43] -> _
    frame False {
      n14 = Create Folder(path (use dialog)=w42, error in=w41) -> (created path=w40:path, error out=w39:errorcluster)  [unwired: 1 in, 1 out]
    }
    frame True {
    }
  }
  n15 = Build Path(base path=w17, name or relative path="Parameter data.xml" ("이름 또는 상대 경로")) -> (appended path=w16:path)
  n16 = while {
    tunnel: "cmd" -> [w49]
    shift-right: [w47] -> w2
    shift-left: "error in" -> [w48]
    shift-right: [w46] -> _
    shift-left: w16 -> [w45]
    stop <- TRUE stop-if-true
    n17 = case shown="\"save\", 기본" w49 {
      tunnel: w48 -> [w52 w62]
      tunnel: [w55 w61] -> w47
      tunnel: [w54 w59] -> w46
      tunnel: w45 -> [w53 w60]
      frame "save", Default {
        n18 = Flatten To XML(anything="Config") -> (xml string=w57:string)
        n19 = call-poly <vilib>:"Write to XML File.vi"("error in (no error)"=w52, "XML Input"=w57, "XML File Path"=w53) -> ("error out"=w55:errorcluster, "XML String"=→"XML String":string, "XML File Path(duplicate)"=w54:path)  [unwired: 6 in]
      }
      frame "load" {
        n20 = call-poly <vilib>:"Read From XML File.vi"("error in (no error)"=w62, "XML File Path"=w60) -> ("error out"=w63:errorcluster, "XML Elements"=w58:string, "XML File Path(duplicate)"=w59:path)  [unwired: 7 in]
        n21 = Unflatten From XML(xml string=w58, type=T1 {"Lower Cut-Off"=0.5, "Vacuum Trigger level"=20.0, "state settings"={"method"=enum."histogram", "histogram size"=0, "histogram method"=enum."mode", "reserved"=0.0}, "SPA-300 Setting"={"Bonding force (g)"=0.0, "Bonding time (ms)"=0.0, "Pickup force (g)"=0.0, "Pickup time (ms)"=0.0, "Speed"=enum."Slow"}, "sensor file"=path ""} ("Config"), error in (no error)=w63) -> (value=→"var":T1, error out=w61:errorcluster)
        n22 = local write "XML String"(w58) -> ()
      }
    }
  }
  "error out" <- w2
